vi "Obtain.vi"(7 "Timer in":refnum<class "Timer.lvclass">, 8 "error in (no error)":errorcluster, 9 "UserEvent":T1, 10 "TimePeroid(ms)":i64, 11 "Name":string) -> (0 "error out":errorcluster, 3 "Timer out":refnum<class "Timer.lvclass">)   [LabVIEW 2017, in "TimerEngine.lvlib" / "Timer.lvclass"]
uses:
  Timer.lvclass
  _Typedef/Timer-UserEvent.ctl
  Timer.lvclass/Timer.ctl
  TimerEngine.lvclass
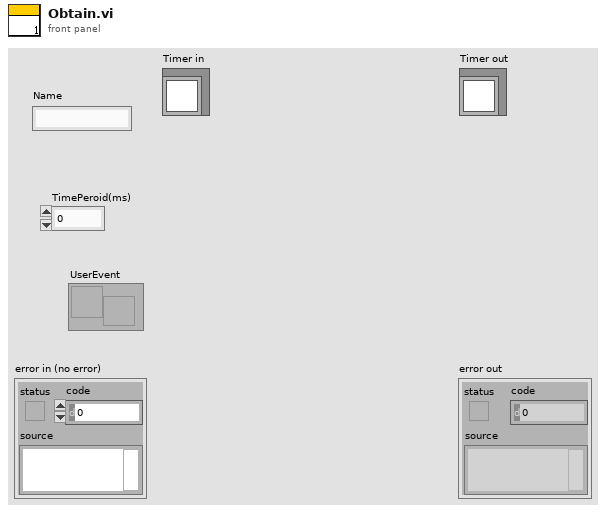
[diagram p1: front panel]
types:
  T1 = typedef "TimerEngine.lvlib/TimerEngine.lvclass/Timer-UserEvent.ctl" = refnum<user-event>
  T2 = typedef "TimerEngine.lvlib/TimerEngine.lvclass/Timer-Userevent.ctl" = refnum<user-event>
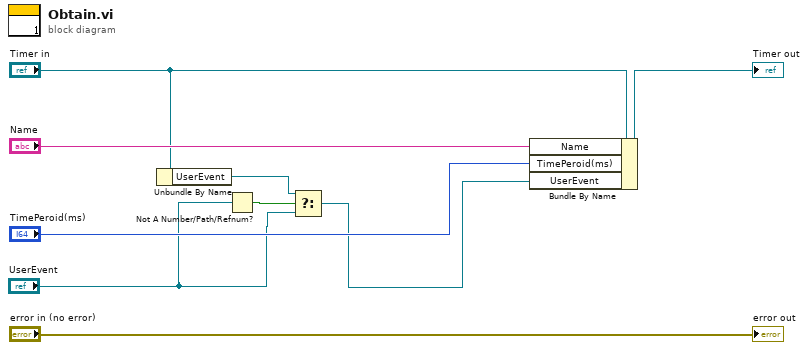
[diagram p0: block diagram]
diagram:
  n1 = Unbundle By Name("Timer in") -> ("UserEvent"=w1:T2)
  n2 = Not A Number/Path/Refnum?(number/path/refnum="UserEvent") -> (NaN/Path/Refnum?=w5:bool)
  n3 = Select(t=w1, s=w5, f="UserEvent") -> (s? t:f=w3:T1)
  n4 = Bundle By Name(cluster="Timer in", "Name"="Name", "TimePeroid(ms)"="TimePeroid(ms)", "UserEvent"=w3) -> (→"Timer out":refnum<class "Timer.lvclass">)
  "error out" <- "error in (no error)"
